vi "PKDAQAppendBlockDataCont.vi"(9 "Run Summary":T1, 10 "Block Data":T2) -> (0 "Transmission":dbl, 2 "Run Summary Out":T1)   [LabVIEW 2013]
uses:
  ctl/SummaryData.ctl
  ctl/BlockData.ctl
  <vilib>/Analysis/baseanly.llb/Mean (DBL).vi
  <vilib>/Analysis/NI_AALBase.lvlib
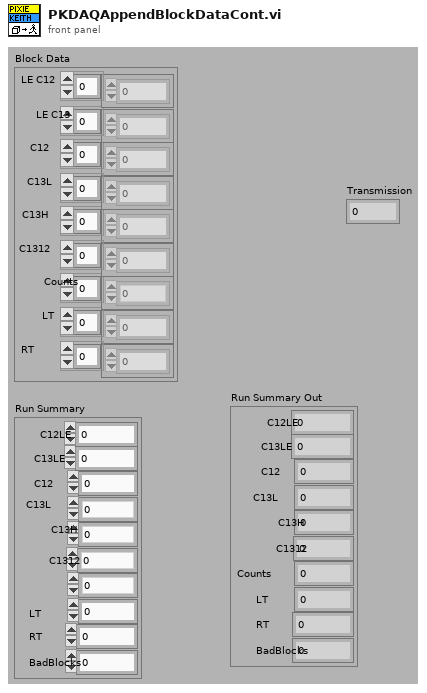
[diagram p1: front panel]
types:
  T1 = typedef "SummaryData.ctl" = cluster{"C12LE":dbl, "C13LE":dbl, "C12":dbl, "C13L":dbl, "C13H":dbl, "C1312":dbl, "Counts":u32, "LT":dbl, "RT":dbl, "BadBlocks":u8}
  T2 = typedef "BlockData.ctl" = cluster{"LE C12":dbl[], "LE C13":dbl[], "C12":dbl[], "C13L":dbl[], "C13H":dbl[], "C1312":dbl[], "Counts":u32[], "LT":dbl[], "RT":dbl[]}
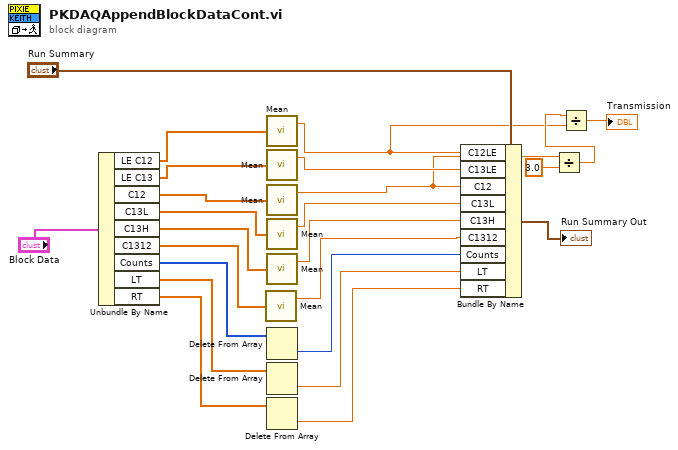
[diagram p0: block diagram]
diagram:
  n1 = Unbundle By Name("Block Data") -> ("LE C12"=w7:dbl[], "LE C13"=w6:dbl[], "C12"=w22:dbl[], "C13L"=w21:dbl[], "C13H"=w20:dbl[], "C1312"=w10:dbl[], "Counts"=w17:u32[], "LT"=w15:dbl[], "RT"=w13:dbl[])
  n2 = call-poly <vilib>:"Mean.vi"("X"=w10) -> ("mean"=w9:dbl)  [unwired: 1 out]
  n3 = call-poly <vilib>:"Mean.vi"("X"=w7) -> ("mean"=w2:dbl)  [unwired: 1 out]
  n4 = call-poly <vilib>:"Mean.vi"("X"=w6) -> ("mean"=w8:dbl)  [unwired: 1 out]
  n5 = call-poly <vilib>:"Mean.vi"("X"=w22) -> ("mean"=w5:dbl)  [unwired: 1 out]
  n6 = call-poly <vilib>:"Mean.vi"("X"=w21) -> ("mean"=w19:dbl)  [unwired: 1 out]
  n7 = call-poly <vilib>:"Mean.vi"("X"=w20) -> ("mean"=w18:dbl)  [unwired: 1 out]
  n8 = Delete From Array(array=w17) -> (deleted portion=w16:u32)  [unwired: 2 in, 1 out]
  n9 = Delete From Array(array=w15) -> (deleted portion=w14:dbl)  [unwired: 2 in, 1 out]
  n10 = Delete From Array(array=w13) -> (deleted portion=w12:dbl)  [unwired: 2 in, 1 out]
  n11 = Bundle By Name(cluster="Run Summary", "C12LE"=w2, "C13LE"=w8, "C12"=w5, "C13L"=w19, "C13H"=w18, "C1312"=w9, "Counts"=w16, "LT"=w14, "RT"=w12) -> (→"Run Summary Out":T1)
  n12 = Divide(x=w5, y=3.0) -> (x/y=w3:dbl)
  n13 = Divide(x=w3, y=w2) -> (x/y=→"Transmission":dbl)
